vi "AddXmiHeader.vi"(8 "error in (no error)":errorcluster, 10 "XmiContent":string, 11 "DiagramName":string) -> (0 "error out":errorcluster, 2 "XmiDocument":string)   [LabVIEW 2012, in "Graph.lvclass"]
uses:
  <resource>/Framework/Providers/Open_GDS/UML/Graph_class/Graph.lvclass
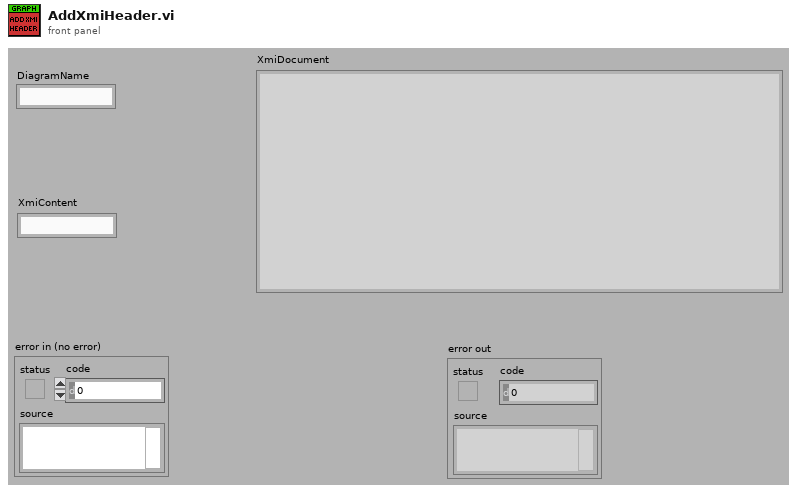
[diagram p1: front panel]
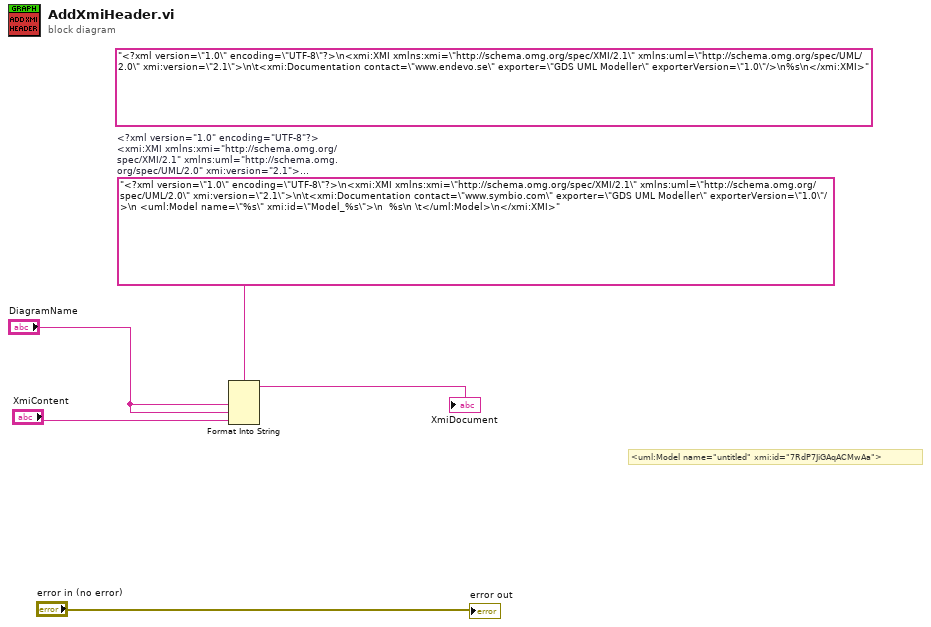
[diagram p0: block diagram]
diagram:
  (unwired) "<?xml version=\"1.0\" encoding=\"UTF-8\"?>\n<xmi:XMI xmlns:xmi=\"http://schema.omg.org/spec/XMI/2.1\" xmlns:uml=\"http://schema.omg.org/spec/UML/2.0\" xmi:version=\"2.1\">\n\t<xmi:Documentation contact=\"www.endevo.se\" exporter=\"GDS UML Modeller\" exporterVersion=\"1.0\"/>\n%s\n</xmi:XMI>"
  w3 = "<?xml version=\"1.0\" encoding=\"UTF-8\"?>\n<xmi:XMI xmlns:xmi=\"http://schema.omg.org/spec/XMI/2.1\" xmlns:uml=\"http://schema.omg.org/spec/UML/2.0\" xmi:version=\"2.1\">\n\t<xmi:Documentation contact=\"www.symbio.com\" exporter=\"GDS UML Modeller\" exporterVersion=\"1.0\"/>\n <uml:Model name=\"%s\" xmi:id=\"Model_%s\">\n  %s\n \t</uml:Model>\n</xmi:XMI>"  # <?xml version="1.0" encoding="UTF-8"?> <xmi:XMI xmlns:xmi="http://schema.omg.org/spec/XMI/2.1" xmlns:uml="http://schema.omg.org/spec/UML/2.0" xmi:version="2.1"> 	<xmi:Documentation contact="www.symbio.com" exporter="GDS UML Modeller" exporterVersion="1.0"/>  <uml:Model name="%s" xmi:id="Model_%s">   %s  	</uml:Model> </xmi:XMI>
  # "<uml:Model name=\"untitled\" xmi:id=\"7RdP7JiGAqACMwAa\">"
  n1 = Format Into String(format string=w3, "DiagramName", "DiagramName", "XmiContent") -> (resulting string=→"XmiDocument":string)  [unwired: 2 in, 1 out]
  "error out" <- "error in (no error)"
